vi "Rio_Theta_Motor_Calibration.vi"(8 "error in (no error)":errorcluster) -> (0 "error out":errorcluster, 3 "Theta Sequence & Position":cluster{i32, dbl})   [LabVIEW 2017]
doc: "This VI rotates the Theta axis counter clockwise until a limit switch is triggered. The index of the motor stepping sequence at this point is outputed.\n\nWritten by Stefan Clarkson, Robin Moore & Thomas Quinn 26/02/18."
uses:
  stepper_half_sequence.ctl
  <vilib>/myRIO/Instrument Drivers/Onboard IO/DIO/typedefs/DIO Reference.ctl
  <vilib>/myRIO/Common/Instrument Driver Framework/Utilities/typedefs/myRIO Generic Hardware Reference.ctl
  <vilib>/myRIO/Common/Instrument Driver Framework/Utilities/typedefs/Hardware Version Enum.ctl
  <vilib>/myRIO/Common/Instrument Driver Framework/Utilities/typedefs/myRIO v1.0 Reference.ctl
  <vilib>/myRIO/Common/Instrument Driver Framework/Utilities/typedefs/Generic FPGA Reference.ctl
  <vilib>/myRIO/Common/Instrument Driver Framework/myRIO v1.0/DIO/typedefs/DIO Channels List.ctl
  <vilib>/myRIO/Common/Instrument Driver Framework/myRIO v1.0/DIO/typedefs/DIO Channels Enum.ctl
  <vilib>/userdefined/High Color/nirio_resource_hc.ctl
  <vilib>/myRIO/Common/Instrument Driver Framework/Utilities/vis/Is FPGA Ref Available.vi
  <vilib>/myRIO/Common/Instrument Driver Framework/myRIO v1.0/DIO/vis/myRIO v1.1 Open DIO.vi
  <vilib>/myRIO/Instrument Drivers/Onboard IO/DIO/vis/Read.vi
  <vilib>/myRIO/Instrument Drivers/Onboard IO/DIO/vis/Write.vi
  <vilib>/myRIO/Common/Instrument Driver Framework/Utilities/vis/Validate Channels.vi
  <vilib>/myRIO/Common/Instrument Driver Framework/myRIO v1.0/DIO/vis/myRIO v1.0 Reserve DIO.vi
  <vilib>/myRIO/Common/Instrument Driver Framework/myRIO v1.0/Resource Manager/vis/myRIO v1.0 Reserve Channel List.vi
  <vilib>/myRIO/Common/Instrument Driver Framework/myRIO v1.0/DIO/vis/myRIO v1.0 Build MUX Configuration DIO.vi
  <vilib>/myRIO/Common/Instrument Driver Framework/myRIO v1.0/Resource Manager/vis/myRIO v1.0 Reserve Channel.vi
  <vilib>/myRIO/Common/Instrument Driver Framework/myRIO v1.0/Resource Manager/vis/myRIO v1.0 Unreserve Channel.vi
  <vilib>/myRIO/Common/Instrument Driver Framework/myRIO v1.0/Resource Manager/vis/myRIO v1.0 Create Configuration List.vi
  <vilib>/myRIO/Common/Instrument Driver Framework/myRIO v1.0/Resource Manager/vis/myRIO v1.0 Build Mutex Name.vi
  <vilib>/Utility/VariantDataType/GetNumericInfo.vi
  <vilib>/Utility/error.llb/Error Cluster From Error Code.vi
  <vilib>/myRIO/Common/Instrument Driver Framework/myRIO v1.0/myRIO v1.1 Open.vi
  <vilib>/myRIO/Common/Instrument Driver Framework/Utilities/vis/IO Manager.vi
  <vilib>/myRIO/Common/Instrument Driver Framework/Utilities/vis/Configuration Manager.vi
  <vilib>/myRIO/Common/Instrument Driver Framework/myRIO v1.0/Resource Manager/vis/myRIO v1.0 Configure IO.vi
  <vilib>/myRIO/Common/Instrument Driver Framework/myRIO v1.0/myRIO v1.0 Close.vi
  <vilib>/myRIO/Common/Instrument Driver Framework/myRIO v1.0/DIO/vis/myRIO v1.0 Read DIO.vi
  <vilib>/myRIO/Common/Instrument Driver Framework/myRIO v1.0/DIO/vis/myRIO v1.0 Write DIO.vi
  <vilib>/myRIO/Express VI/Onboard IO/DI/DI Express VI.xnode
  <vilib>/myRIO/Instrument Drivers/Onboard IO/DIO/vis/myRIO DIO Open.xnode
  <vilib>/myRIO/Express VI/Onboard IO/DO/DO Express VI.xnode
  <vilib>/myRIO/Instrument Drivers/Onboard IO/DIO/DIO.lvlib
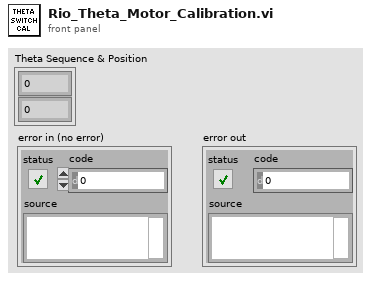
[diagram p1: front panel]
types:
  T1 = typedef "DIO.lvlib/DIO Reference.ctl" = cluster{"myRIO Reference":T2, "DIO Channels List":T6}
  T2 = typedef "myRIO Generic Hardware Reference.ctl" = cluster{"myRIO Model":T3, "myRIO Hardware Reference":T4}
  T3 = typedef "Hardware Version Enum.ctl" = enum16{"Unknown", "myRIO-1900", "myRIO-1950", "roboRIO", "NI ELVIS RIO CM"}
  T4 = typedef "myRIO v1.0 Reference.ctl" = cluster{"Generic FPGA Reference":T5, "Allow multiple opens":bool}
  T5 = typedef "Generic FPGA Reference.ctl" = refnum<k20>
  T6 = typedef "DIO Channels List.ctl" = T7[]
  T7 = typedef "DIO Channels Enum.ctl" = enum16{"Not Connected", "C/DIO0", "C/DIO1", "C/DIO2", "C/DIO3", "C/DIO4", "C/DIO5", "C/DIO6", "C/DIO7", "A/DIO0", "A/DIO1", "A/DIO2", "A/DIO3", "A/DIO4", "A/DIO5", "A/DIO6", "A/DIO7", "A/DIO8", "A/DIO9", "A/DIO10", "A/DIO11", "A/DIO12", "A/DIO13", "A/DIO14", "A/DIO15", "B/DIO0", "B/DIO1", "B/DIO2", "B/DIO3", "B/DIO4", "B/DIO5", "B/DIO6", "B/DIO7", "B/DIO8", "B/DIO9", "B/DIO10", "B/DIO11", "B/DIO12", "B/DIO13", "B/DIO14", "B/DIO15", "LED0", "LED1", "LED2", "LED3", "Button0", "DIO/DIO0", "DIO/DIO1", "DIO/DIO2", "DIO/DIO3", "DIO/DIO4", "DIO/DIO5", "DIO/DIO6", "DIO/DIO7", "DIO/DIO8", "DIO/DIO9", "SPI/CS0", "SPI/CS1", "SPI/CS2", "SPI/CS3", "LED RADIO (Green)", "LED RADIO (Red)", "LED COMM (Green)", "LED COMM (Red)", "LED MODE (Green)", "LED MODE (Red)"}
  T8 = typedef "nirio_resource_hc.ctl" = tag
  T9 = typedef "stepper_half_sequence.ctl" = cluster{i32[]}
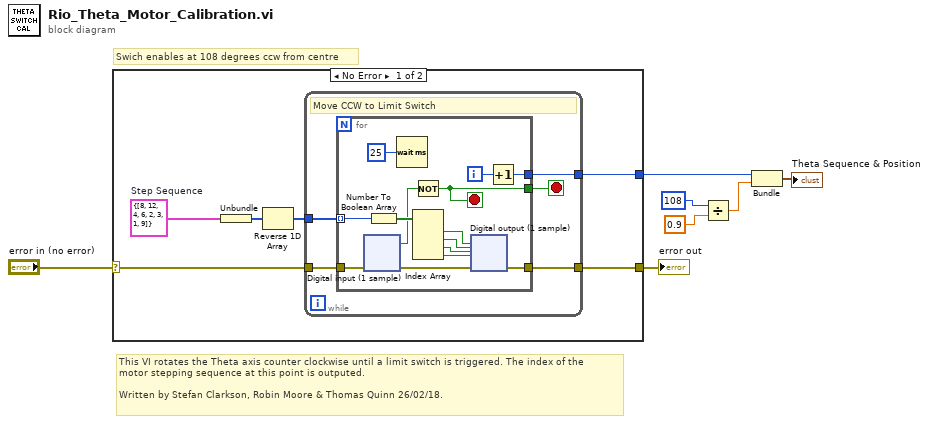
[diagram p0: block diagram]
diagram:
  # "This VI rotates the Theta axis counter clockwise until a limit switch is triggered. The index of the \nmotor stepping sequence at this point is outputed.\n\nWritten by Stefan Clarkson, Robin Moore & Thomas Quinn 26/02/18."
  # "Swich enables at 108 degrees ccw from centre"
  n1 = case shown="No Error" "error in (no error)" {
    selector: "error in (no error)" -> [w8 w106]
    tunnel: [w13 w106] -> w6
    tunnel: [w12 _] -> w3
    frame No Error {
      w10 = T9 {[8, 12, 4, 6, 2, 3, 1, 9]}  # Step Sequence
      n2 = Unbundle(w10) -> (w9:i32[])
      n3 = Reverse 1D Array(array=w9) -> (reversed array=w11:i32[])
      n4 = while {
        tunnel: w11 -> [w15]
        tunnel: [w18] -> w13
        tunnel: w8 -> [w17]
        tunnel: [w16] -> w12
        stop <- w14 stop-if-true
        # "Move CCW to Limit Switch"
        n5 = for {
          tunnel: w15 -> [w25] mode=indexing
          tunnel: [w28] -> w18
          tunnel: w17 -> [w26]
          tunnel: [w21] -> w16
          tunnel: [w22] -> w14
          i -> [w20]
          stop <- w22 stop-if-true
          n6 = xnode ("Digital input (1 sample)")("error in (no error)"=w26) -> ("error out"=w19:errorcluster, "Theta Limit Switch (A/DIO13 (Pin 26))"=w27:bool)
          n7 = Number To Boolean Array(number=w25) -> (Boolean array=w32:bool[])
          n8 = Wait (ms)(milliseconds to wait=u32 25) -> ()  [unwired: 1 out]
          n9 = Not(x=w27) -> (.not. x?=w22:bool)
          n10 = Index Array(array=w32) -> (element #1=w31:bool, element #2=w24:bool, element #3=w23:bool, element #4=w30:bool)  [unwired: 4 in]
          n11 = xnode ("Digital output (1 sample)")("error in (no error)"=w19, "0 (A/DIO0 (Pin 11))"=w31, "1 (A/DIO1 (Pin 13))"=w24, "2 (A/DIO2 (Pin 15))"=w23, "3 (A/DIO3 (Pin 17))"=w30) -> ("error out"=w28:errorcluster)
          n12 = Increment(x=w20) -> (x+1=w21:i32)
        }
      }
    }
    frame Error {
    }
  }
  "error out" <- w6
  n13 = Divide(x=108, y=0.9) -> (x/y=w2:dbl)
  n14 = Bundle(w3, w2) -> (→"Theta Sequence & Position":cluster{i32, dbl})  [unwired: 1 in]
